vi "GetOperatingState.vi"(8 "error in":errorcluster, 9 "index":i32, 10 "operating states":variant, 11 "data group":string) -> (0 "error out":errorcluster, 3 "operating state":T1)   [LabVIEW 2017, in "OpState.lvlib"]
uses:
  <vilib>/addons/InsightCM/Devices/Shared/Common/OpState/OpState.lvlib
  <vilib>/addons/InsightCM/Devices/Shared/Common/OpState/controls/TriggerOperatingState.ctl
  <vilib>/addons/InsightCM/MessageBus/Base/controls/KeyValuePair.ctl
  <vilib>/addons/InsightCM/Devices/Shared/Common/Trigger/controls/TriggerCondition.ctl
  <vilib>/addons/InsightCM/MessageBus/Base/controls/Condition.ctl
  <vilib>/addons/InsightCM/Devices/Shared/Common/Trigger/Trigger.lvlib
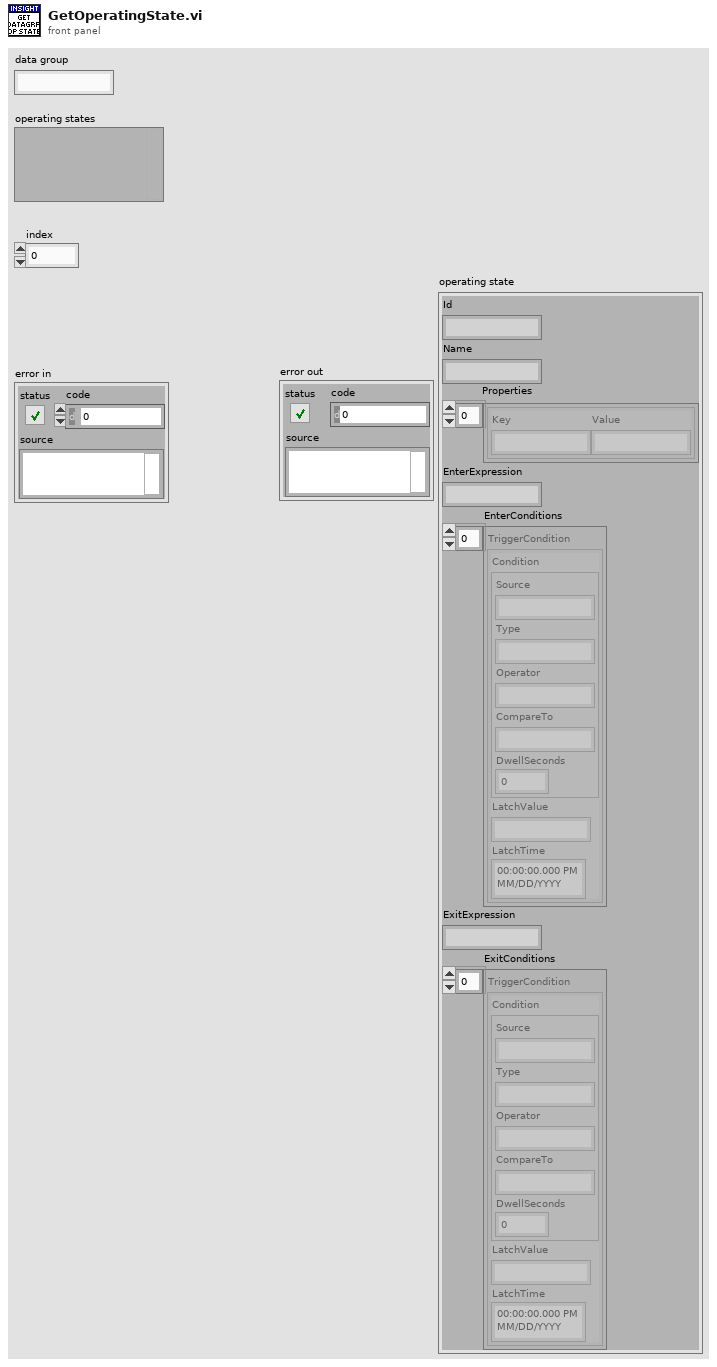
[diagram p1: front panel]
types:
  T1 = typedef "OpState.lvlib/TriggerOperatingState.ctl" = cluster{"Id":string, "Name":string, "Properties":T2[], "EnterExpression":string, "EnterConditions":T3[], "ExitExpression":string, "ExitConditions":T3[]}
  T2 = typedef "KeyValuePair.ctl" = cluster{"Key":string, "Value":string}
  T3 = typedef "Trigger.lvlib/TriggerCondition.ctl" = cluster{"Condition":T4, "LatchValue":string, "LatchTime":timestamp}
  T4 = typedef "Condition.ctl" = cluster{"Source":string, "Type":string, "Operator":string, "CompareTo":string, "DwellSeconds":dbl}
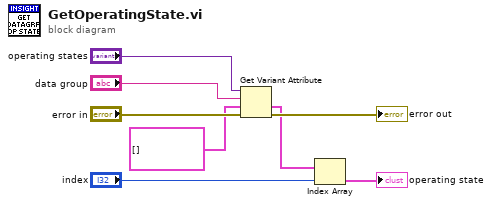
[diagram p0: block diagram]
diagram:
  n1 = Get Variant Attribute(Variant="operating states", name="data group", default value (empty Variant)=T1[] [] ("OperatingStates"), error in="error in") -> (value=w3:T1[], error out=→"error out":errorcluster)  [unwired: 2 out]
  n2 = Index Array(array=w3, index="index") -> (element=→"operating state":T1)
